vi "KDH_EX3Task4_1-23-17.vi"() -> ()   [LabVIEW 2014, in "Harris_MacMaster_4th_LEGORobotics_11-29-16.lvrbt"]
uses:
  Harris_MacMaster_4th_LEGORobotics_11-29-16.lvrbt
panel:
  out "XY Graph":cluster{"X":dbl, "Y":dbl}[](graph)
  out "Waveform Graph":dbl[][](graph)
  out "Sweep Chart":cluster{dbl, dbl}(graph)
  out "Scope Chart":cluster{dbl, dbl}(graph)
  out "Strip Chart":cluster{dbl, dbl}(graph)
  out "Moving Average":dbl
  in  "stop":bool
  out "Random Number":dbl
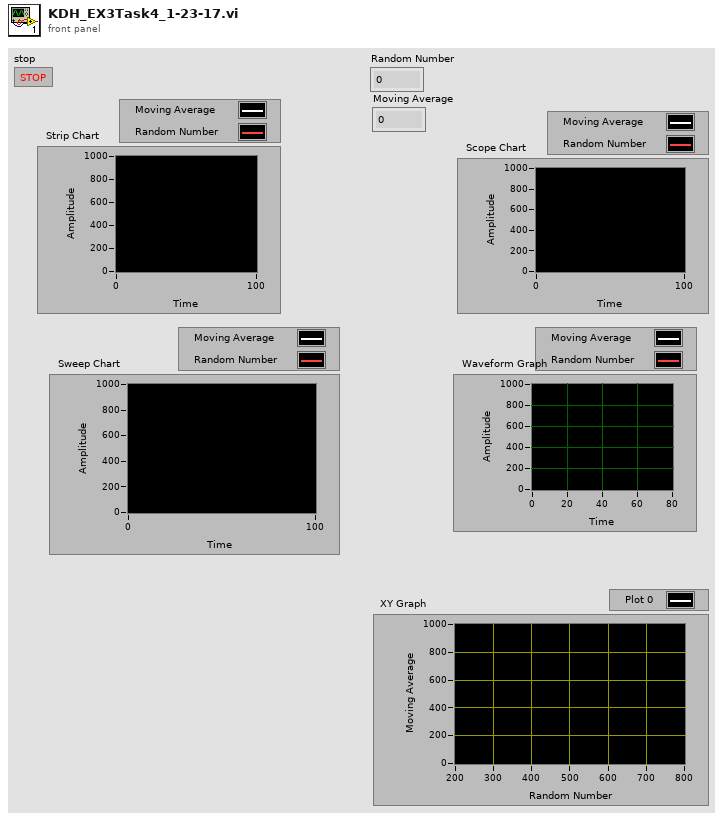
[diagram p1: front panel]
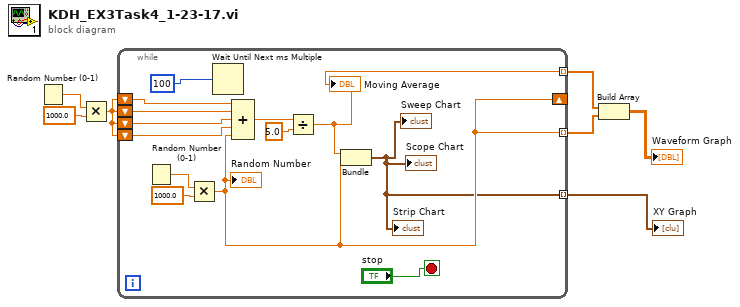
[diagram p0: block diagram]
diagram:
  n1 = Random Number (0-1)() -> (number: 0 to 1=w6:dbl)
  n2 = Multiply(x=w6, y=1000.0) -> (x*y=w5:dbl)
  n3 = while {
    shift-right: [w9] -> _
    shift-left: w5 -> [w17]
    shift-left: w5 -> [w16]
    shift-left: w5 -> [w15]
    shift-left: w5 -> [w14]
    tunnel: [w10] -> w4 mode=indexing
    tunnel: [w9] -> w2 mode=indexing
    tunnel: [w8] -> w1 mode=indexing
    stop <- "stop" stop-if-true
    n4 = Random Number (0-1)() -> (number: 0 to 1=w19:dbl)
    n5 = Multiply(x=w19, y=1000.0) -> (x*y=w9:dbl)
    "Random Number" <- w9
    n6 = Wait Until Next ms Multiple(millisecond multiple=u32 100) -> ()  [unwired: 1 out]
    n7 = Compound Arithmetic op=ADD(w17, w16, w15, w14, w9) -> (w12:dbl)
    n8 = Divide(x=w12, y=5.0) -> (x/y=w10:dbl)
    "Moving Average" <- w10
    n9 = Bundle(w10, w9) -> (w8:cluster{dbl, dbl})  [unwired: 1 in]
    "Strip Chart" <- w8
    "Scope Chart" <- w8
    "Sweep Chart" <- w8
  }
  "XY Graph" <- w1
  n10 = Build Array(w4, w2) -> (→"Waveform Graph":dbl[][])
